vi "ConfigInstr.vi"(6 "InstrumentName":string, 7 "VisaRes":refnum<visa-resource-name>="COM1", 8 "error in (no error)":errorcluster caption="entrée d'erreur (pas d'erreur)", 9 "FirstClassInst":bool, 10 "Function":string, 11 "OR77200 In":refnum<class "OR77200.lvclass"> caption="DNL_LabVIEW Object in") -> (0 "error out":errorcluster caption="sortie d'erreur", 3 "OR77200 Out":refnum<class "OR77200.lvclass"> caption="DNL_LabVIEW Object out")   [LabVIEW 2019, in "OR77200.lvclass"]
uses:
  OR77200.lvclass
  C:/Programmes Labview/LabScanV1A/DevicesClass/BaseDevice/BaseDevice.lvclass
  OR77200_Func.ctl
  OR77200.lvclass/OR77200.ctl
  BaseDevice/BaseDevice.lvclass/BaseDevice.ctl
  BaseDevice/Accessor/SetShowInstrNm.vi
panel:
  in  "OR77200_Func":T1
  out "VisaRes":refnum<visa-resource-name>
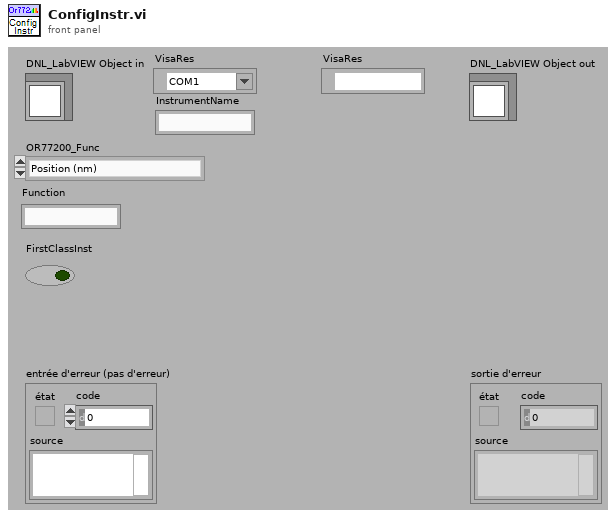
[diagram p1: front panel]
types:
  T1 = typedef "OR77200.lvclass/OR77200_Func.ctl" = enum16{"Position (nm)"}
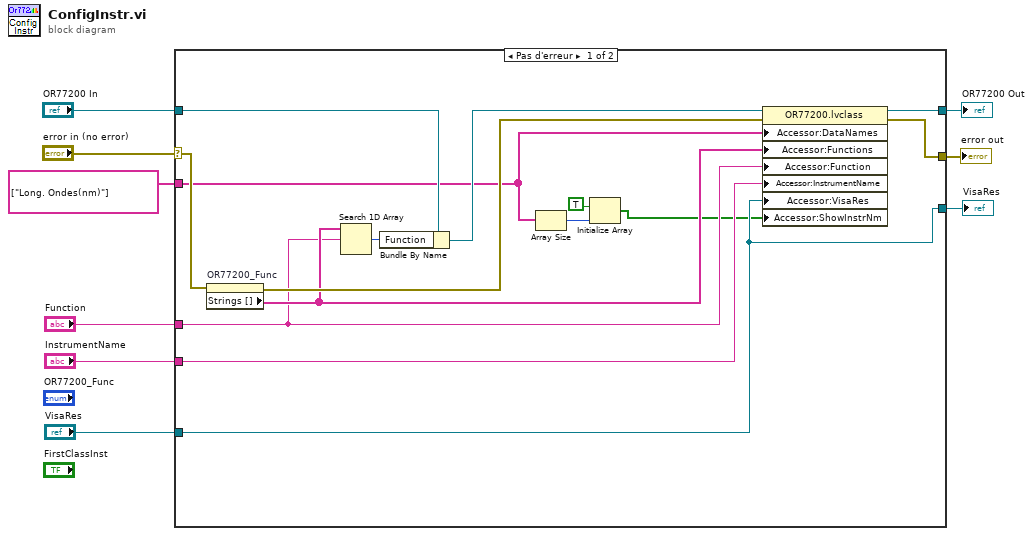
[diagram p0: block diagram]
diagram:
  n1 = case shown="Pas d'erreur" "error in (no error)" {
    selector: "error in (no error)" -> [w20 w26]
    tunnel: [w15 w26] -> w8
    tunnel: "OR77200 In" -> [w23 w25]
    tunnel: [w18 w25] -> w6
    tunnel: string[] ["Long. Ondes(nm)"] -> [w11 _]
    tunnel: [w14 _] -> w4
    tunnel: "Function" -> [w17 _]
    tunnel: "VisaRes" -> [w14 _]
    tunnel: "InstrumentName" -> [w16 _]
    frame No Error {
      n2 = property on="OR77200_Func" class="Énum (strict)"(error in=w20) -> (error out=w21:errorcluster, "Strings []"=w19:string[])  [unwired: 1 in, 1 out]
      n3 = Search 1D Array(1D array=w19, element=w17) -> (index of element=w24:i32)  [unwired: 1 in]
      n4 = Bundle By Name(cluster=w23, "Function"=w24) -> (w22:refnum<class "OR77200.lvclass">)
      n5 = Array Size(array=w11) -> (size(s)=w13:i32)
      n6 = Initialize Array(TRUE, w13) -> (w10:bool[])
      n7 = property class="OR77200.lvclass"(reference=w22, error in=w21, "Accessor:DataNames"=w11, "Accessor:Functions"=w19, "Accessor:Function"=w17, "Accessor:InstrumentName"=w16, "Accessor:VisaRes"=w14, "Accessor:ShowInstrNm"=w10) -> (reference out=w18:refnum<class "OR77200.lvclass">, error out=w15:errorcluster)
    }
    frame Error {
    }
  }
  "error out" <- w8
  "OR77200 Out" <- w6
  "VisaRes" <- w4
